vi "Test Device.vi"() -> ()   [LabVIEW 2015]
doc: "Example VI that demonstrates all library features."
uses:
  Test Device/Test Device.lvclass
  <vilib>/plasmapper/PL BlackBox Modbus Client/PL BlackBox Modbus Client.lvclass
  <vilib>/plasmapper/PL DNS Client/PL DNS Client.lvlib
panel:
  in  "read graph":bool
  out "graph":sgl[](graph)
  out "inputs":T1
  in  "parameters":T2
  in  "save configuration":bool
  out "TD":refnum<class "Test Device.lvclass">
  in  "read configuration":bool=TRUE
  out "uid":string
  out "firmware":string
  out "hardware":string
  out "device name":string
  in  "interface":enum32{"serial", "TCP"}(tab)
  in  "serial settings":T3={"port"="", "protocol"=enum."RTU", "address"=1, "baud rate"=115200, "data bits"=8, "parity"=2, "stop bits"=10, "flow control"=0} {"flow control" items=["None", "XON/XOFF", "RTS/CTS", "XON/XOFF & RTS/CTS", "DTR/DSR", "XON/XOFF & DTR/DSR"]; "stop bits" items=["1.0"=10, "1.5"=15, "2.0"=20]; "parity" items=["None", "Odd", "Even", "Mark", "Space"]}
  in  "TCP settings":T4={"ip address"="192.168.1.1", "port"=502, "station address"=255}
  in  "find service":bool
  in  "service name":string="TestDevice"
  out "error":errorcluster
  in  "stop":bool
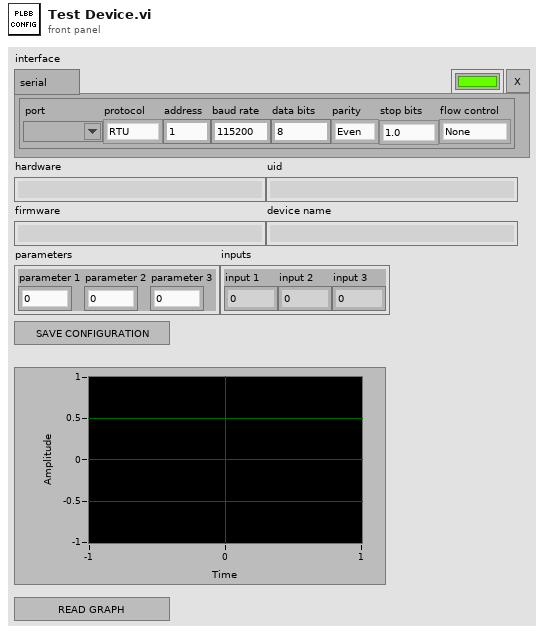
[diagram p1: front panel]
types:
  T1 = cluster{"input 1":u16, "input 2":u16, "input 3":u16}
  T2 = cluster{"parameter 1":u16, "parameter 2":u16, "parameter 3":u16}
  T3 = cluster{"port":refnum<visa-resource-name>, "protocol":enum16{"RTU", "ASCII"}, "address":u8, "baud rate":u32, "data bits":u16, "parity":u16, "stop bits":u16, "flow control":u16}
  T4 = cluster{"ip address":string, "port":u16, "station address":u8}
  T5 = cluster{"hardware":cluster{"name":string, "version":cluster{"major":u16, "minor":u16, "patch":u16}, "uid":string}, "firmware":cluster{"name":string, "version":cluster{"major":u16, "minor":u16, "patch":u16}}, "number of hardware interfaces":u16, "number of servers":u16}
  T6 = cluster{"instance name":string, "hostname":string, "address":string, "port":u16, "priority":u16, "weight":u16, "additional information":cluster{"name":string, "value":string}[]}[]
  T7 = cluster{"instance name":string, "hostname":string, "address":string, "port":u16, "priority":u16, "weight":u16, "additional information":cluster{"name":string, "value":string}[]}
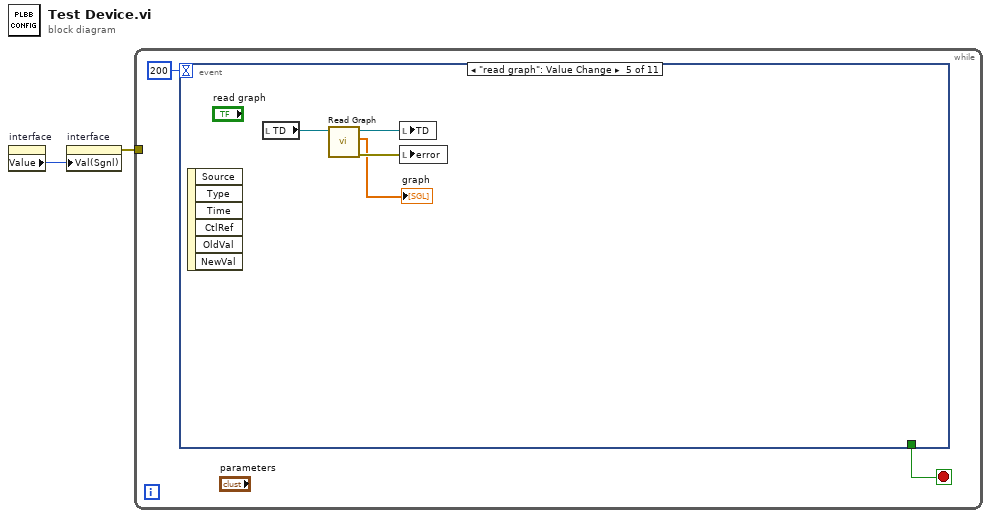
[diagram p0: block diagram]
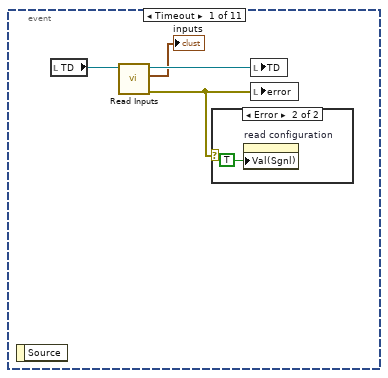
[diagram p2: hidden frame]
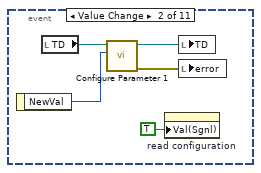
[diagram p4: hidden frame]
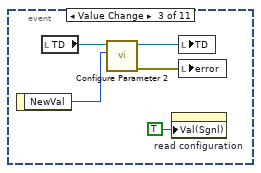
[diagram p5: hidden frame]
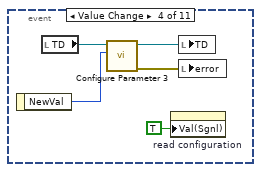
[diagram p6: hidden frame]
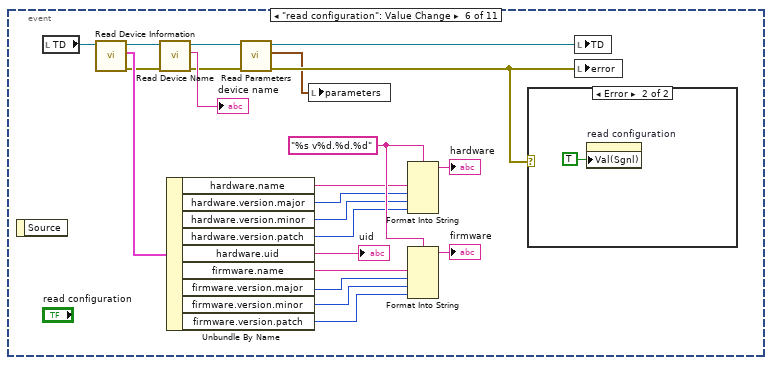
[diagram p7: hidden frame]
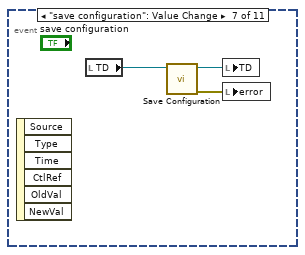
[diagram p9: hidden frame]
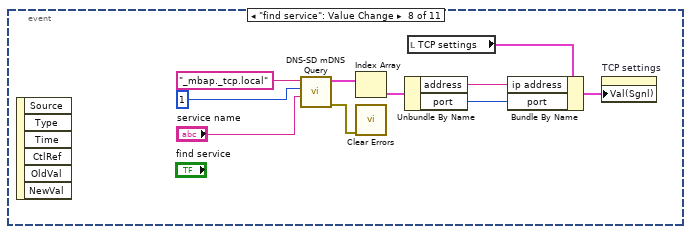
[diagram p10: hidden frame]
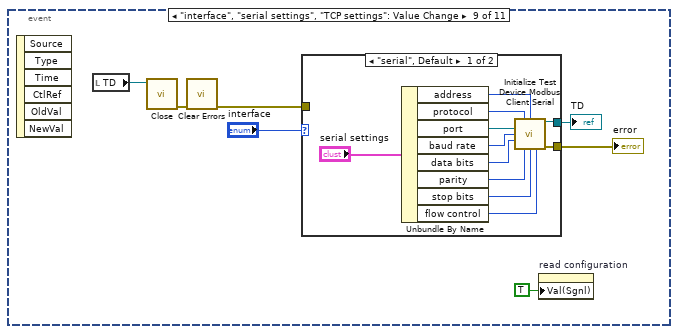
[diagram p11: hidden frame]
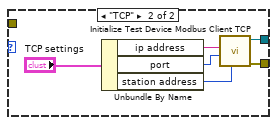
[diagram p12: hidden frame]
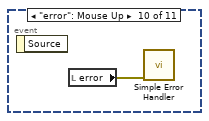
[diagram p13: hidden frame]
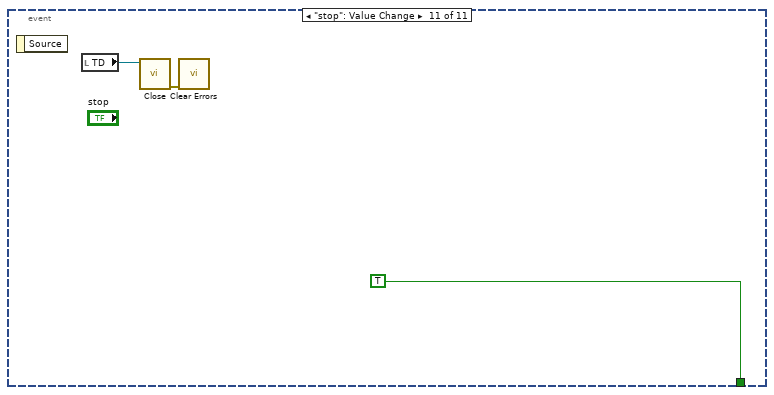
[diagram p14: hidden frame]
diagram:
  n1 = property on="interface" class="TabCtl (strict)"() -> ("Value"=w2:enum32{"serial", "TCP"})  [unwired: 2 in, 2 out]
  n2 = property on="interface" class="TabCtl (strict)"("Val(Sgnl)"=w2) -> (error out=w1:errorcluster)  [unwired: 2 in, 1 out]
  n3 = while {
    tunnel: w1 -> [_]
    stop <- w3 stop-if-true
    n4 = event shown="[4] \"read graph\": Value Change" {
      selector: _ -> [_ _ _ _ _ _ _ _ _ _ _]
      dyn-events: _ -> [_ _ _ _ _ _ _ _ _ _ _]
      timeout: 200 -> [_ _ _ _ _ _ _ _ _ _ _]
      tunnel: [_ _ _ _ _ _ _ _ _ _ TRUE ("stop")] -> w3
      event Timeout {
        n5 = event-data() -> ()  [unwired: 1 in, 1 out]
        n6 = local read "TD"() -> (w8:refnum<class "Test Device.lvclass">)
        n7 = call "Read Inputs.vi"("PLBB in"=w8) -> ("error out"=w6:errorcluster, "inputs"=→"inputs":T1, "PLBB out"=w7:refnum<class "Test Device.lvclass">)  [unwired: 8 in]
        n8 = case shown="Error" w6 {
          frame No Error {
          }
          frame Error {
            n9 = property on="read configuration" class="Bool (strict)"("Val(Sgnl)"=TRUE ("Value (Signaling)")) -> ()  [unwired: 2 in, 2 out]
          }
        }
        n10 = local write "TD"(w7) -> ()
        n11 = local write "error"(w6) -> ()
      }
      event "parameters.parameter 1": Value Change {
        n12 = event-data() -> ("NewVal"=w11:u16)  [unwired: 1 in]
        n13 = local read "TD"() -> (w12:refnum<class "Test Device.lvclass">)
        n14 = call "Configure Parameter 1.vi"("value"=w11, "PLBB in"=w12) -> ("error out"=w14:errorcluster, "PLBB out"=w13:refnum<class "Test Device.lvclass">)  [unwired: 8 in]
        n15 = property on="read configuration" class="Bool (strict)"("Val(Sgnl)"=TRUE ("Value (Signaling)")) -> ()  [unwired: 2 in, 2 out]
        n16 = local write "TD"(w13) -> ()
        n17 = local write "error"(w14) -> ()
      }
      event "parameters.parameter 2": Value Change {
        n18 = event-data() -> ("NewVal"=w16:u16)  [unwired: 1 in]
        n19 = local read "TD"() -> (w17:refnum<class "Test Device.lvclass">)
        n20 = call "Configure Parameter 2.vi"("value"=w16, "PLBB in"=w17) -> ("error out"=w19:errorcluster, "PLBB out"=w18:refnum<class "Test Device.lvclass">)  [unwired: 8 in]
        n21 = property on="read configuration" class="Bool (strict)"("Val(Sgnl)"=TRUE ("Value (Signaling)")) -> ()  [unwired: 2 in, 2 out]
        n22 = local write "TD"(w18) -> ()
        n23 = local write "error"(w19) -> ()
      }
      event "parameters.parameter 3": Value Change {
        n24 = event-data() -> ("NewVal"=w21:u16)  [unwired: 1 in]
        n25 = local read "TD"() -> (w22:refnum<class "Test Device.lvclass">)
        n26 = call "Configure Parameter 3.vi"("value"=w21, "PLBB in"=w22) -> ("error out"=w24:errorcluster, "PLBB out"=w23:refnum<class "Test Device.lvclass">)  [unwired: 8 in]
        n27 = property on="read configuration" class="Bool (strict)"("Val(Sgnl)"=TRUE ("Value (Signaling)")) -> ()  [unwired: 2 in, 2 out]
        n28 = local write "TD"(w23) -> ()
        n29 = local write "error"(w24) -> ()
      }
      event "read graph": Value Change {
        n30 = event-data() -> ()  [unwired: 1 in, 6 out]
        n31 = local read "TD"() -> (w28:refnum<class "Test Device.lvclass">)
        n32 = call "Read Graph.vi"("PLBB in"=w28) -> ("error out"=w26:errorcluster, "graph"=→"graph":sgl[], "PLBB out"=w27:refnum<class "Test Device.lvclass">)  [unwired: 8 in]
        n33 = local write "TD"(w27) -> ()
        n34 = local write "error"(w26) -> ()
      }
      event "read configuration": Value Change {
        w48 = "%s v%d.%d.%d" ("format string")
        n35 = event-data() -> ()  [unwired: 1 in, 1 out]
        n36 = local read "TD"() -> (w50:refnum<class "Test Device.lvclass">)
        n37 = call <vilib>:"Read Device Information.vi"("PLBB in"=w50) -> ("error out"=w35:errorcluster, "device information"=w49:T5, "PLBB out"=w36:refnum<class "Test Device.lvclass">)  [unwired: 8 in]
        n38 = call <vilib>:"Read Device Name.vi"("error in (no error)"=w35, "PLBB in"=w36) -> ("error out"=w32:errorcluster, "device name"=→"device name":string, "PLBB out"=w33:refnum<class "Test Device.lvclass">)  [unwired: 7 in]
        n39 = Unbundle By Name(w49) -> ("hardware.name"=w47:string, "hardware.version.major"=w46:u16, "hardware.version.minor"=w45:u16, "hardware.version.patch"=w44:u16, "hardware.uid"=→"uid":string, "firmware.name"=w43:string, "firmware.version.major"=w42:u16, "firmware.version.minor"=w41:u16, "firmware.version.patch"=w40:u16)
        n40 = call "Read Parameters.vi"("error in (no error)"=w32, "PLBB in"=w33) -> ("error out"=w31:errorcluster, "parameters"=w29:T2, "PLBB out"=w30:refnum<class "Test Device.lvclass">)  [unwired: 7 in]
        n41 = local write "parameters"(w29) -> ()
        n42 = Format Into String(format string=w48, w47, w46, w45, w44) -> (resulting string=→"hardware":string)  [unwired: 2 in, 1 out]
        n43 = Format Into String(format string=w48, w43, w42, w41, w40) -> (resulting string=→"firmware":string)  [unwired: 2 in, 1 out]
        n44 = case shown="Error" w31 {
          frame No Error {
          }
          frame Error {
            n45 = property on="read configuration" class="Bool (strict)"("Val(Sgnl)"=TRUE ("Value (Signaling)")) -> ()  [unwired: 2 in, 2 out]
          }
        }
        n46 = local write "TD"(w30) -> ()
        n47 = local write "error"(w31) -> ()
      }
      event "save configuration": Value Change {
        n48 = event-data() -> ()  [unwired: 1 in, 6 out]
        n49 = local read "TD"() -> (w53:refnum<class "Test Device.lvclass">)
        n50 = call <vilib>:"Save Configuration.vi"("PLBB in"=w53) -> ("error out"=w54:errorcluster, "PLBB out"=w52:refnum<class "Test Device.lvclass">)  [unwired: 9 in]
        n51 = local write "TD"(w52) -> ()
        n52 = local write "error"(w54) -> ()
      }
      event "find service": Value Change {
        n53 = event-data() -> ()  [unwired: 1 in, 6 out]
        n54 = call <vilib>:"DNS-SD mDNS Query.vi"("instance name (any)"="service name", "max number of instances (all)"=u32 1, "service.domain"="_mbap._tcp.local") -> ("error out"=w61:errorcluster, "service instances"=w60:T6)  [unwired: 7 in]
        n55 = Index Array(array=w60) -> (element=w59:T7)  [unwired: 1 in]
        n56 = call <vilib>:"Clear Errors.vi"("error in (no error)"=w61) -> ()  [unwired: 5 in, 2 out]
        n57 = Unbundle By Name(w59) -> ("address"=w57:string, "port"=w56:u16)
        n58 = local read "TCP settings"() -> (w58:T4)
        n59 = Bundle By Name(cluster=w58, "ip address"=w57, "port"=w56) -> (w55:T4)
        n60 = property on="TCP settings" class="Clust (strict)"("Val(Sgnl)"=w55) -> ()  [unwired: 2 in, 2 out]
      }
      event "interface", "serial settings", "TCP settings": Value Change {
        n61 = event-data() -> ()  [unwired: 1 in, 6 out]
        n62 = local read "TD"() -> (w70:refnum<class "Test Device.lvclass">)
        n63 = call-dynamic "Close.vi"("TD in"=w70) -> ("error out"=w71:errorcluster)  [unwired: 10 in]
        n64 = call <vilib>:"Clear Errors.vi"("error in (no error)"=w71) -> ("error out"=w68:errorcluster)  [unwired: 5 in, 1 out]
        n65 = case shown="\"serial\", Default" "interface" {
          tunnel: [w82 w88] -> w66
          tunnel: [w81 w87] -> w67
          tunnel: w68 -> [_ _]
          frame "serial", Default {
            n66 = Unbundle By Name("serial settings") -> ("address"=w73:u8, "protocol"=w74:enum16{"RTU", "ASCII"}, "port"=w76:refnum<visa-resource-name>, "baud rate"=w75:u32, "data bits"=w77:u16, "parity"=w78:u16, "stop bits"=w79:u16, "flow control"=w80:u16)
            n67 = call "Initialize Test Device Modbus Client Serial.vi"("protocol (RTU)"=w74, "station address (1)"=w73, "port"=w76, "baud rate (115200)"=w75, "data bits (8)"=w77, "parity (even)"=w78, "stop bits (1.0)"=w79, "flow control (none)"=w80) -> ("PLBB out"=w82:refnum<class "Test Device.lvclass">, "error out"=w81:errorcluster)  [unwired: 6 in]
          }
          frame "TCP" {
            n68 = Unbundle By Name("TCP settings") -> ("ip address"=w85:string, "port"=w84:u16, "station address"=w83:u8)
            n69 = call "Initialize Test Device Modbus Client TCP.vi"("station address (255)"=w83, "port (502)"=w84, "ip address"=w85) -> ("error out"=w87:errorcluster, "TD out"=w88:refnum<class "Test Device.lvclass">)  [unwired: 7 in]
          }
        }
        "error" <- w67
        "TD" <- w66
        n70 = property on="read configuration" class="Bool (strict)"("Val(Sgnl)"=TRUE ("Value (Signaling)")) -> ()  [unwired: 2 in, 2 out]
      }
      event "error": Mouse Up {
        n71 = event-data() -> ()  [unwired: 1 in, 1 out]
        n72 = local read "error"() -> (w89:errorcluster)
        n73 = call <vilib>:"Simple Error Handler.vi"("error in (no error)"=w89) -> ()  [unwired: 4 in, 5 out]
      }
      event "stop": Value Change {
        n74 = event-data() -> ()  [unwired: 1 in, 1 out]
        n75 = local read "TD"() -> (w90:refnum<class "Test Device.lvclass">)
        n76 = call-dynamic "Close.vi"("TD in"=w90) -> ("error out"=w91:errorcluster)  [unwired: 10 in]
        n77 = call <vilib>:"Clear Errors.vi"("error in (no error)"=w91) -> ()  [unwired: 5 in, 2 out]
      }
    }
  }
